vi "Build Report String.vi"(8 "error in (no error)":errorcluster, 10 "Result":T1, 11 "Window Action in":refnum<class "Window Action.lvclass">) -> (0 "error out":errorcluster, 2 "Report String":string, 3 "Window Action out":refnum<class "Window Action.lvclass">)   [LabVIEW 2020, in "MacroAssert.lvlib" / "Window Action.lvclass"]
doc: "Builds a string using <B>Step</B> and <B>Result</B> to be included in a report."
uses:
  Window Action.lvclass
  CTLs/Result.ctl
  CTLs/Outcome.ctl
  Action Step/Action Step.lvclass
  MacroAssert.lvlib
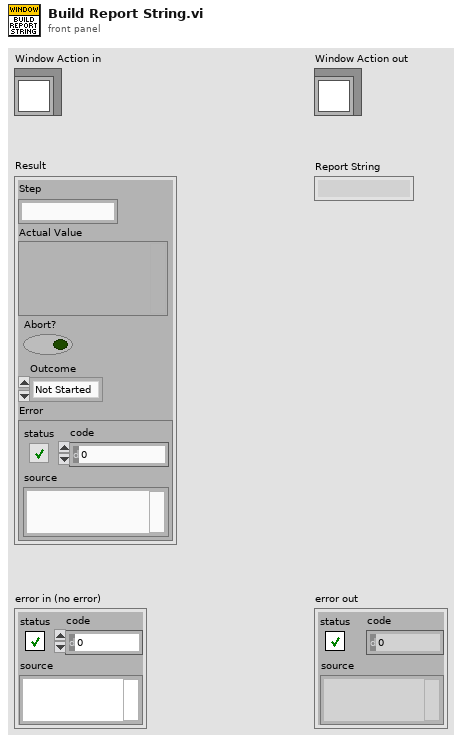
[diagram p1: front panel]
types:
  T1 = typedef "MacroAssert.lvlib/Result.ctl" = cluster{"Step":string, "Actual Value":variant, "Abort?":bool, "Outcome":T2, "Error":errorcluster}
  T2 = typedef "MacroAssert.lvlib/Outcome.ctl" = enum16{"Not Started", "Skipped", "Pass", "Fail", "Complete", "Error", "Auto Abort", "User Abort"}
  T3 = typedef "MacroAssert.lvlib/Window Action.lvclass/Window Action Type.ctl" = enum16{"Maximize Window", "Restore Window", "Minimize Window", "Close Window", "Bring Window to Front", "Send Window to Back"}
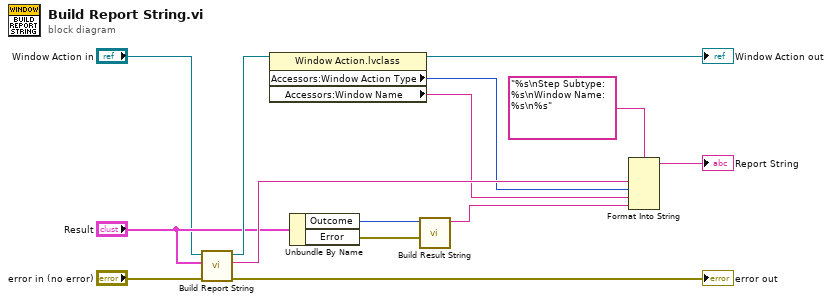
[diagram p0: block diagram]
diagram:
  n1 = call-parent "Build Report String.vi"("error in (no error)"="error in (no error)", "Result"="Result", "Step in"="Window Action in") -> ("error out"=→"error out":errorcluster, "Report String"=w9:string, "Step out"=w10:refnum<class "Window Action.lvclass">)  [unwired: 6 in]
  n2 = property class="Window Action.lvclass"(reference=w10) -> (reference out=→"Window Action out":refnum<class "Window Action.lvclass">, "Accessors:Window Action Type"=w8:T3, "Accessors:Window Name"=w2:string)  [unwired: 1 in, 1 out]
  n3 = Unbundle By Name("Result") -> ("Outcome"=w12:T2, "Error"=w14:errorcluster)
  n4 = call "Build Result String.vi"("Error"=w14, "Outcome"=w12) -> ("Result String"=w11:string)  [unwired: 9 in]
  n5 = Format Into String(format string="%s\nStep Subtype: %s\nWindow Name: %s\n%s", w9, w8, w2, w11) -> (resulting string=→"Report String":string)  [unwired: 2 in, 1 out]
